vi "Read Limit Test Results.vi"(8 "error in (no error)":errorcluster, 11 "Freq Sweet Result in":refnum<class "Freq Sweep Result.lvclass">) -> (0 "error out":errorcluster, 2 "Limit Test Results":cluster{dbl[], dbl[]}[](array[cluster])=[{[1000.0, 9166.666666666668, 17333.333333333336, 25500.0, 33666.66666666667, 41833.333333333336, 50000.0], [0.8109999999999999, 0.7375, 0.6639999999999999, 0.5905, 0.5169999999999999, 0.44349999999999995, 0.37]}, {[1000.0, 9166.666666666668, 17333.333333333336, 25500.0, 33666.66666666667, 41833.333333333336, 50000.0], [0.7727256581908878, 0.7031032017391705, 0.5983315439720234, 0.5084307021460196, 0.4381322995151595, 0.3914920131543004, 0.35634281183887034]}, {[1000.0, 9166.666666666668, 17333.333333333336, 25500.0, 33666.66666666667, 41833.333333333336, 50000.0], [0.6910000000000001, 0.6174999999999999, 0.544, 0.4705, 0.39699999999999996, 0.32349999999999995, 0.25]}], 3 "Freq Sweet Result out":refnum<class "Freq Sweep Result.lvclass">)   [LabVIEW 2013, in "Frequency Measurement.lvlib" / "Freq Sweep Result.lvclass"]
uses:
  Freq Sweep Result.lvclass
  Freq Sweep Result.lvclass/Freq Sweep Result.ctl
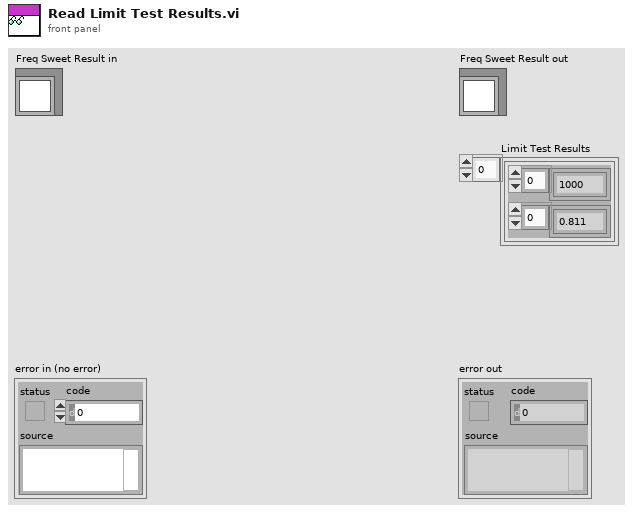
[diagram p1: front panel]
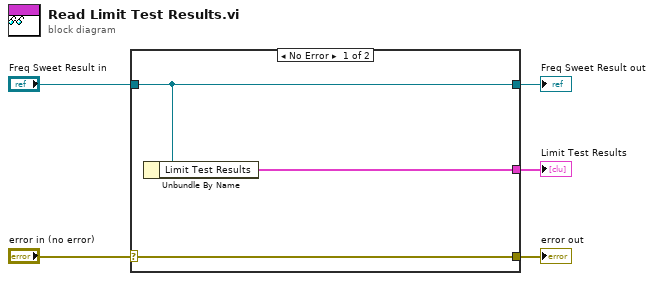
[diagram p0: block diagram]
diagram:
  n1 = case shown="No Error" "error in (no error)" {
    selector: "error in (no error)" -> [w8 w9]
    tunnel: [w8 w9] -> w4
    tunnel: [w7 w10] -> w2
    tunnel: "Freq Sweet Result in" -> [w7 w10]
    tunnel: [w6 _] -> w1
    frame No Error {
      n2 = Unbundle By Name(w7) -> ("Limit Test Results"=w6:cluster{dbl[], dbl[]}[])
    }
    frame Error {
    }
  }
  "error out" <- w4
  "Freq Sweet Result out" <- w2
  "Limit Test Results" <- w1
